vi "Spectrometer Control Panel (No Objects).vi"(8 "error in (no error)":errorcluster) -> (0 "error out":errorcluster)   [LabVIEW 2012]
uses:
  JY-SPEX-TRIAX/controls.llb/Turret Position (TRIAX).ctl
  JY-SPEX-TRIAX/controls.llb/Monochromator System Number.ctl
  JY-SPEX-TRIAX/controls.llb/Mirror Position.ctl
  <vilib>/Utility/error.llb/DialogType.ctl
  JY-SPEX-TRIAX/controls.llb/Slits.ctl
  JY-SPEX-TRIAX/JY-SPEX-TRIAX.lvlib
panel:
  in  "VISA Resource Name":refnum<visa-resource-name>="GPIB0::1::INSTR"
  out "Cluster Out":T4
  in  "Cluster In":T4
  out "?":bool
  out "Title 2":string="Spectrometer Control Program"
  in  "Select Grating":T3
  out "Construct":bool
  out "Init":T5
  out "Status":string
  in  "Shutter":bool
  in  "Set Mirror":bool
  in  "Exit Mirror Pos":bool=TRUE
  in  "Exit":bool
  out "Ready (when flashing)":bool
  out "Slits Open?":bool
  in  "Close Slits":bool
  in  "stepsize":dbl[unit]
  in  "Optimize":bool
  out "groovedensity":dbl[unit] caption="Groove Density"
  out "blazewave":dbl[unit] caption="Blaze Wavelength"
  in  "Set Turret":bool
  out "Title":string="Spectrometer Control Program"
  in  "Reset":bool
  out "Current Wavelength":dbl[unit]
  in  "Target Wavelength":dbl[unit]=4.0000000000000003e-07 min=0.0 max=1.4000000000000001e-06 step=1.0000000000000002e-10
  in  "Jump To Wavelength":bool
  in  "Set Slits":bool
  out "currentlat":dbl[unit] format="%#_6f"
  out "currentaxial":dbl[unit] format="%#_6f"
  in  "gotolat":dbl[unit] min=0.0 max=0.0022 step=1e-05
  in  "gotoaxial":dbl[unit] min=0.0 max=0.0022 step=1e-05 format="%#_6f"
  # "Initialization"
  # "Wavelength Control"
  # "Slit Widths"
  # "Turret and Other Specs"
  # "Target"
  # "Current"
  # "AXIAL/CCD"
  # "LATERAL/PMT"
  # "Axial Entrance"
  # "Lateral Exit"
  # "(will round to nearest step size - 2 µm)"
  # "Grooves/mm       Blaze           Cal Offset\nGrating A           1200           500 nm            -35571\nGrating B           1200           750 nm            -38317\nGrating C             600         1000 nm           -40000 (??)"
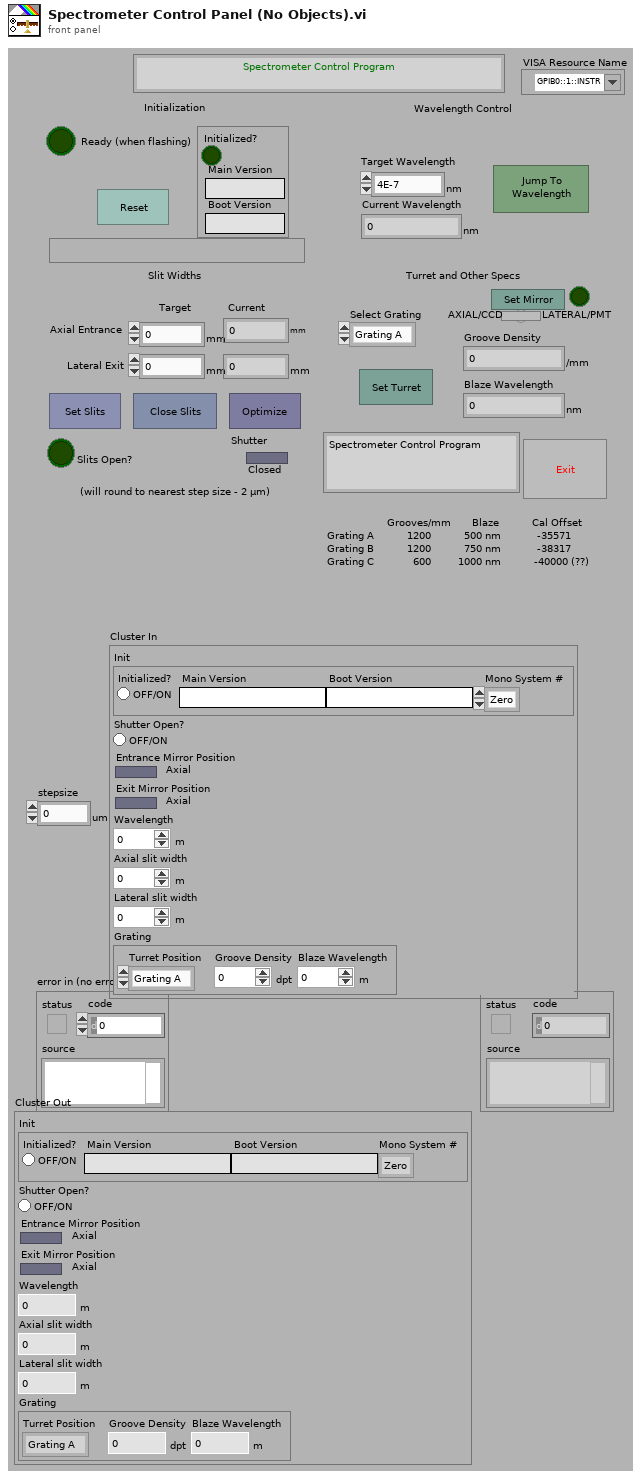
[diagram p1: front panel]
types:
  T1 = typedef "JY-SPEX-TRIAX.lvlib/Monochromator System Number.ctl" = enum16{"Zero", "One"}
  T2 = typedef "JY-SPEX-TRIAX.lvlib/Mirror Position.ctl" = bool
  T3 = typedef "JY-SPEX-TRIAX.lvlib/Turret Position (TRIAX).ctl" = enum16{"Grating A", "Grating B", "Grating C"}
  T4 = cluster{"Init":cluster{"Initialized?":bool, "Main Version":string, "Boot Version":string, "Mono System #":T1}, "Shutter Open?":bool, "Entrance Mirror Position":T2, "Exit Mirror Position":T2, "Wavelength":dbl[unit], "Axial slit width":dbl[unit], "Lateral slit width":dbl[unit], "Grating":cluster{"Turret Position":T3, "Groove Density":dbl[unit], "Blaze Wavelength":dbl[unit]}}
  T5 = cluster{"Initialized?":bool, "Main Version":string, "Boot Version":string, "Spectrometer Number":enum16{"Zero", "One"}}
  T6 = typedef "JY-SPEX-TRIAX.lvlib/Slits.ctl" = enum16{"0 (Front/Axial Entrance)", "1 (Side/Lateral Entrance)", "2 (Front/Axial Exit)", "3 (Side/Lateral Exit)"}
  T7 = typedef "DialogType.ctl" = u16
  T8 = cluster{"Initialized?":bool, "Main Version":string, "Boot Version":string, "Mono System #":T1}
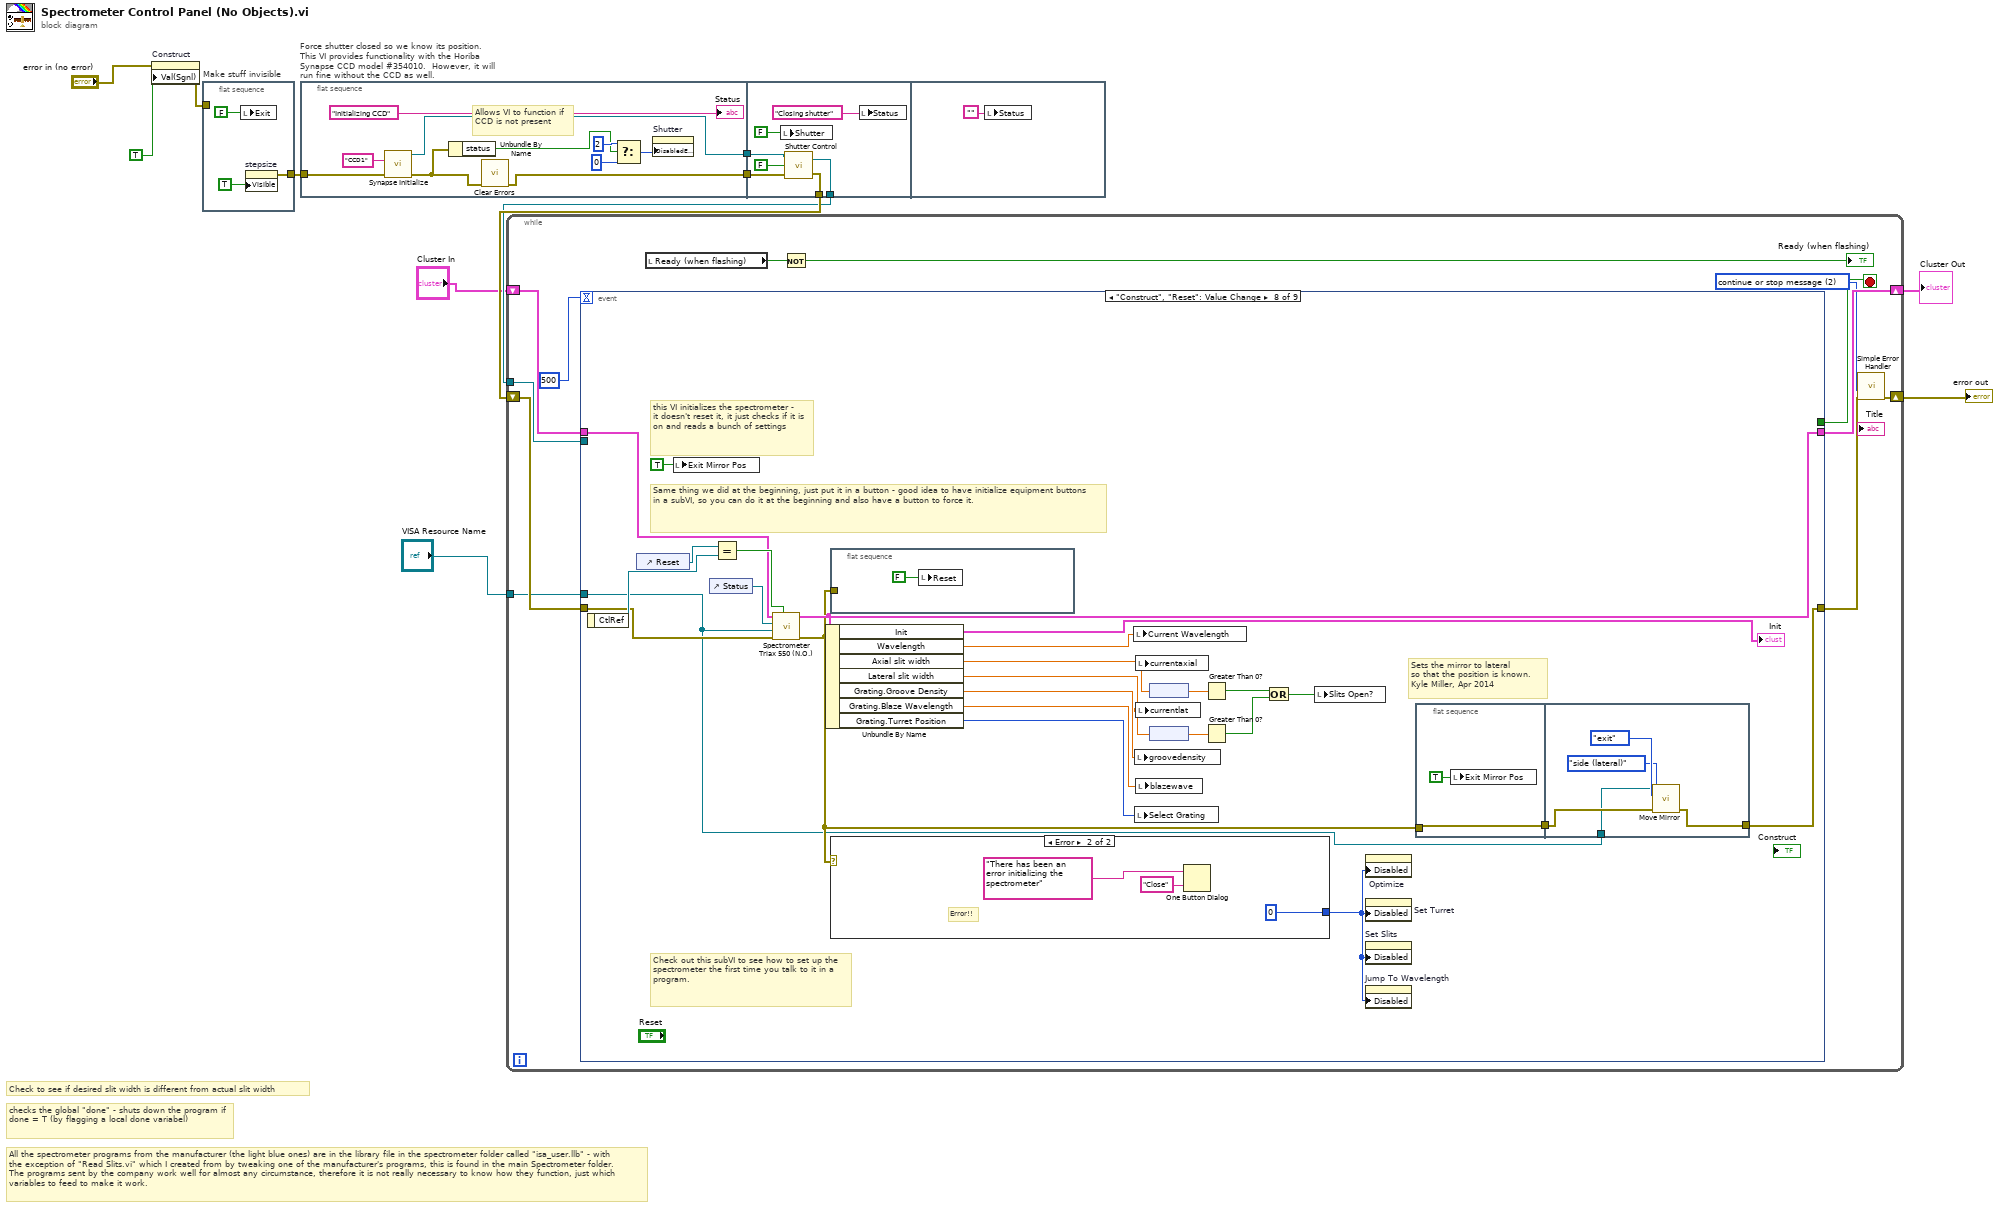
[diagram p0: block diagram]
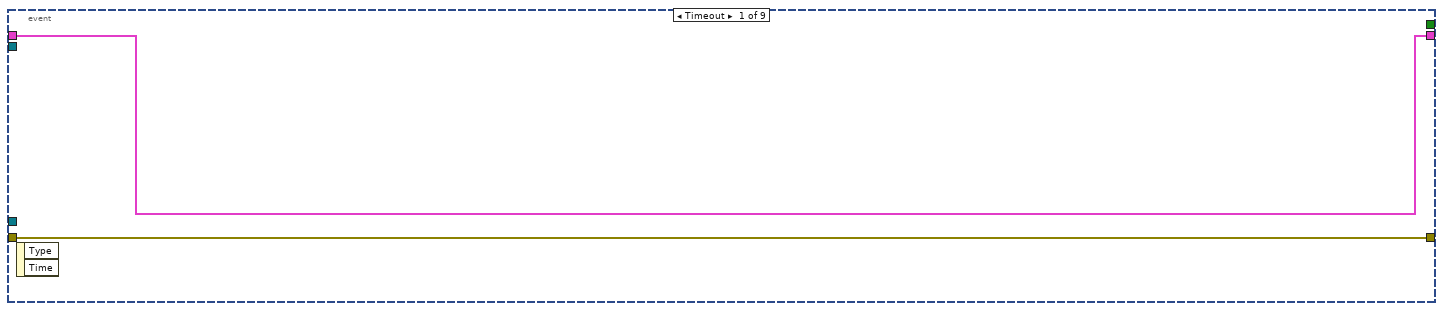
[diagram p2: hidden frame]
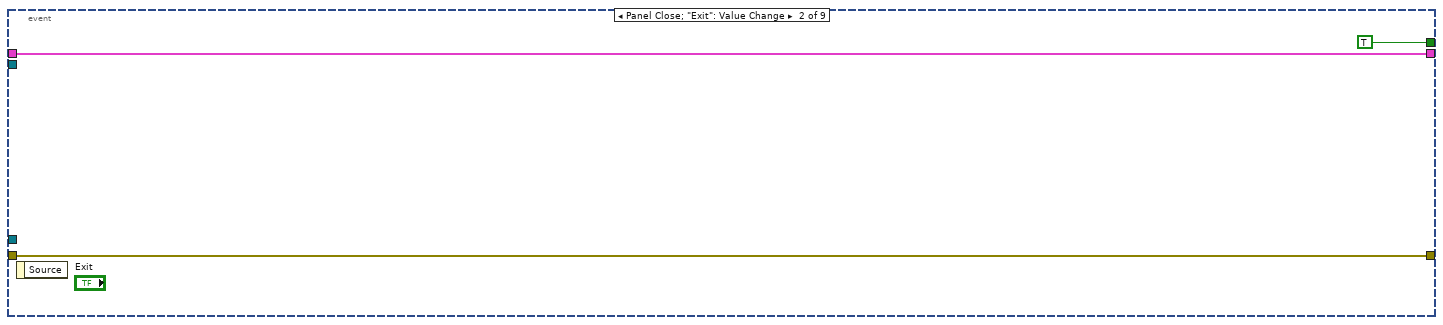
[diagram p3: hidden frame]
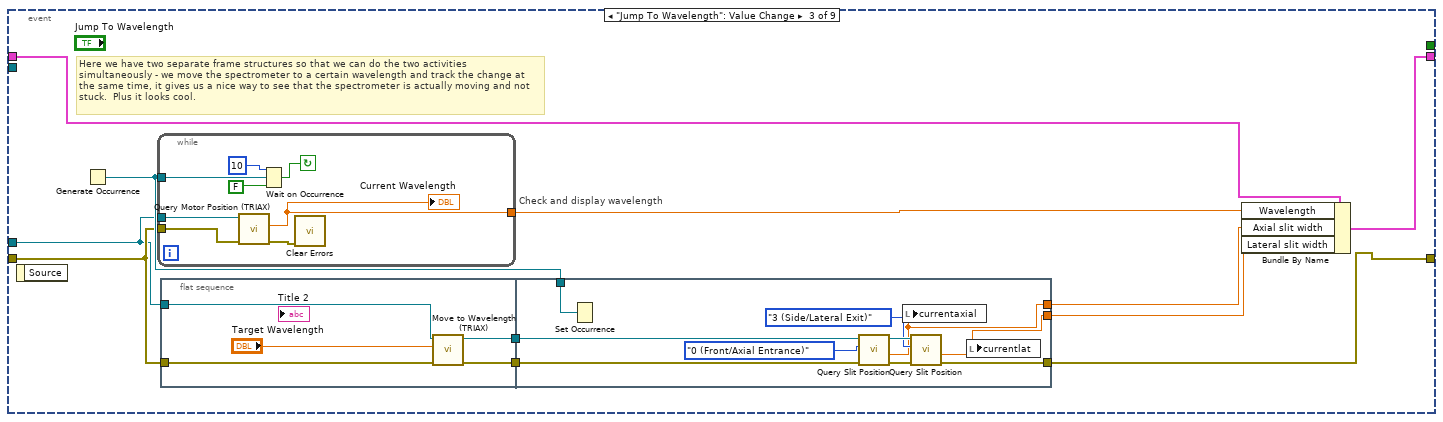
[diagram p4: hidden frame]
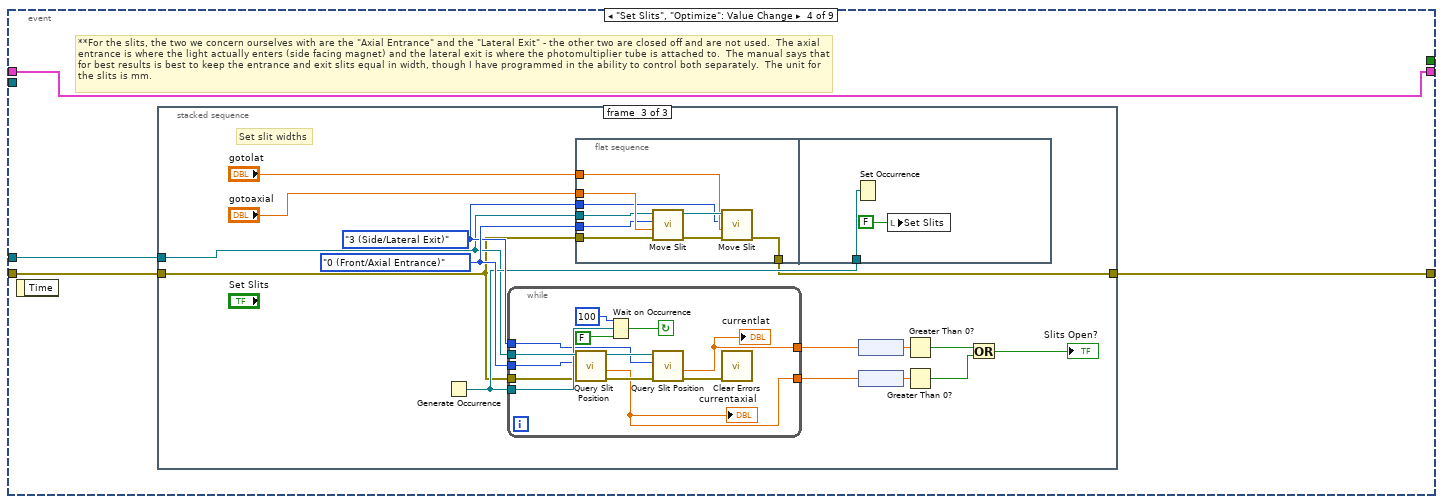
[diagram p5: hidden frame]
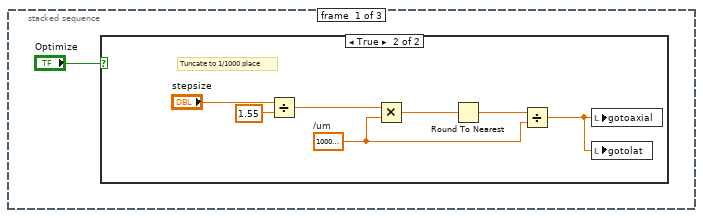
[diagram p6: hidden frame]
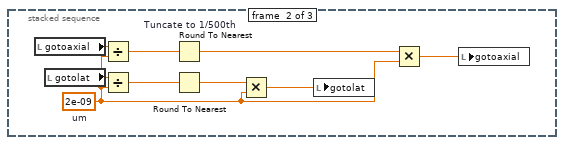
[diagram p8: hidden frame]
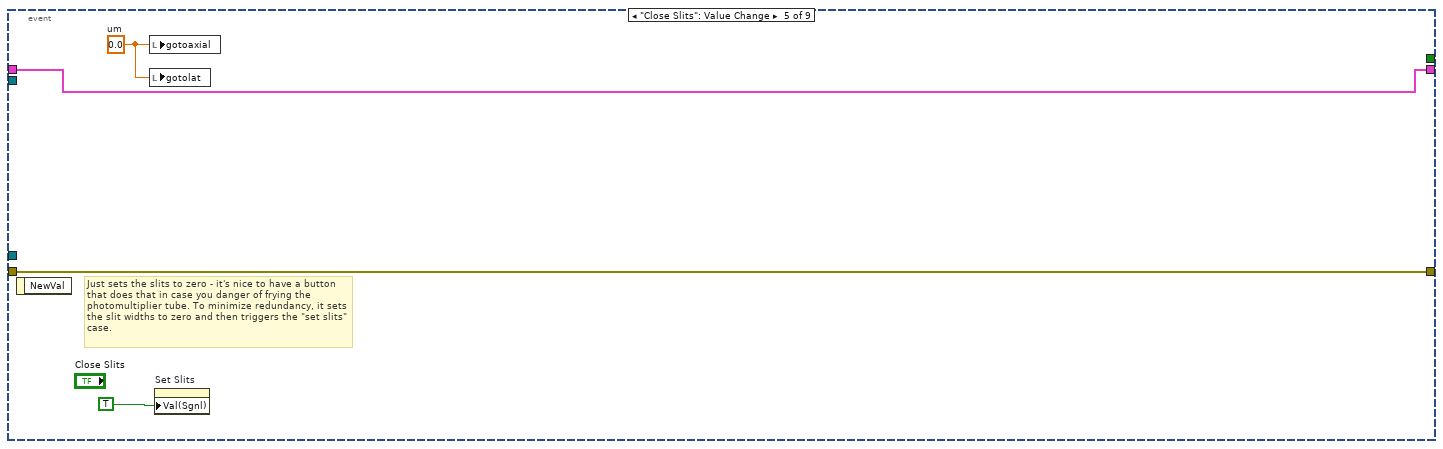
[diagram p9: hidden frame]
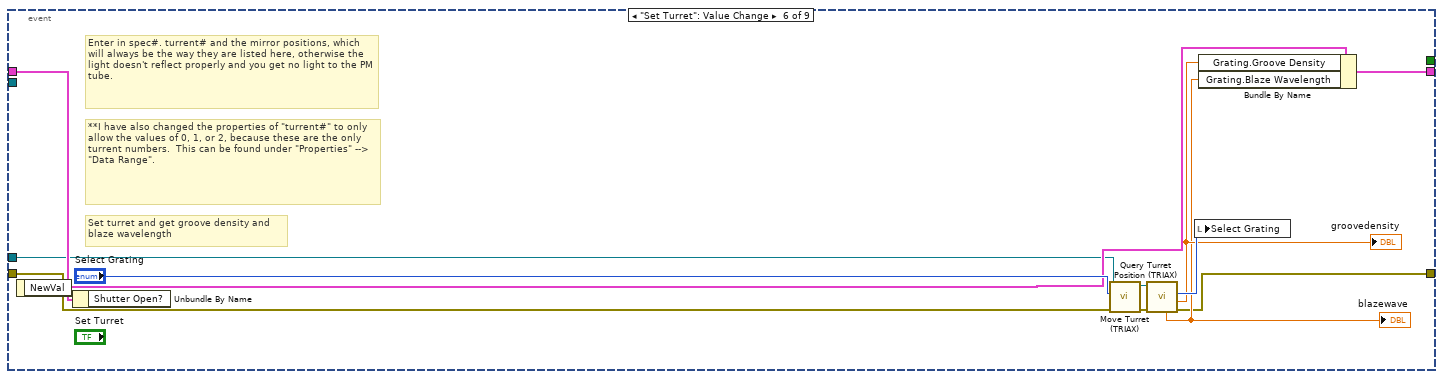
[diagram p10: hidden frame]
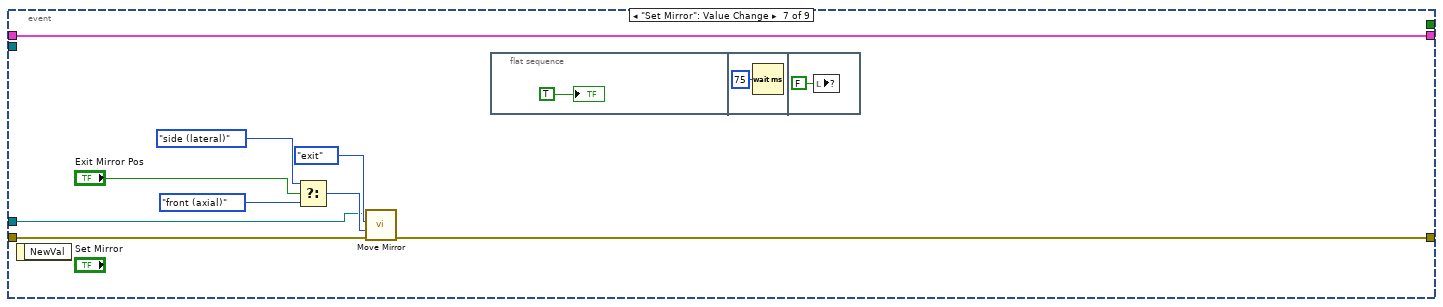
[diagram p11: hidden frame]
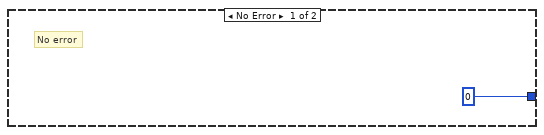
[diagram p12: hidden frame]
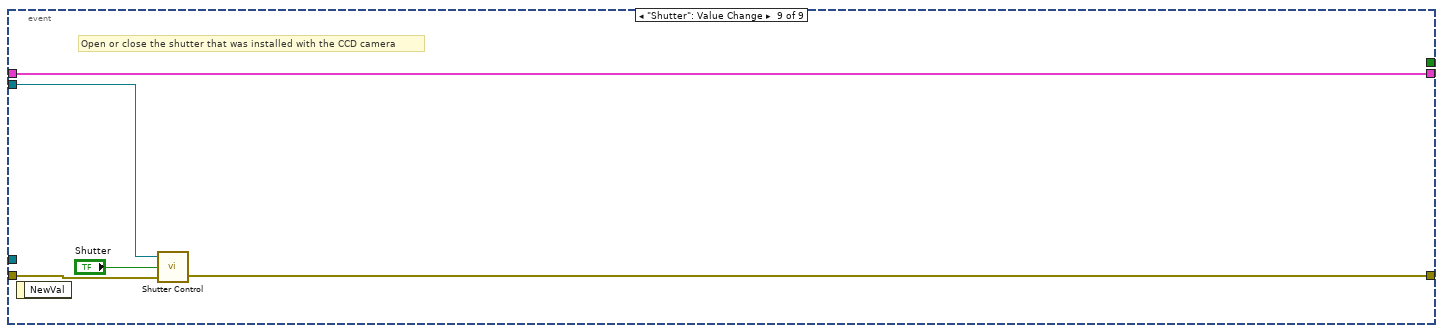
[diagram p13: hidden frame]
diagram:
  # "Check to see if desired slit width is different from actual slit width"
  # "checks the global \"done\" - shuts down the program if done = T (by flagging a local done variabel)"
  # "All the spectrometer programs from the manufacturer (the light blue ones) are in the library file in the spectrometer folder called \"isa_user.llb\" - with the exception of \"Read Slits.vi\" which I created from by tweaking one of the manufacturer's programs, this is found in the main Spectrometer folder.  The programs sent by the company work well for almost any circumstance, therefore it is not really necessary to know how they function, just which variables to feed to make it work."
  n1 = property on="Construct" class="Bool (strict)"(error in="error in (no error)", "Val(Sgnl)"=TRUE ("Value (Signaling)")) -> (error out=w11:errorcluster)  [unwired: 1 in, 1 out]
  n2 = flat-sequence "Make stuff invisible" {
    tunnel: w11 -> [_]
    tunnel: [w14] -> w8
    frame #0 {
      n3 = local write "Exit"(FALSE ("exit")) -> ()
      n4 = property on="stepsize" class="DigNum (strict)"("Visible"=TRUE) -> (error out=w14:errorcluster)  [unwired: 2 in, 1 out]
    }
  }
  n5 = flat-sequence "Force shutter closed so we know its position.  This VI provides functionality with the Horiba Synapse CCD model #354010.  However, it will run fine without the CCD as well." {
    tunnel: w8 -> [w24]
    tunnel: [w18] -> w7
    tunnel: [w22] -> w2
    tunnel: [w30] -> w10
    tunnel: [w29] -> w9
    tunnel: w7 -> [w28]
    tunnel: w2 -> [w27]
    frame #0 {
      # "Allows VI to function if CCD is not present"
      n6 = call "Synapse Initialize.vi"("error in (no error)"=w24, "Unique id"="CCD1") -> ("error out"=w17:errorcluster, "JYCCDLib.IJYCCDReqd"=w22:refnum<k7>)  [unwired: 1 in, 7 out]
      n7 = Unbundle By Name(w17) -> ("status"=w16:bool)
      n8 = call <vilib>:"Clear Errors.vi"("error in (no error)"=w17) -> ("error out"=w18:errorcluster)  [unwired: 6 in]
      n9 = Select(t=2, s=w16, f=0) -> (s? t:f=w19:i32)
      n10 = property on="Shutter" class="Bool (strict)"("DisabledEnum"=w19) -> ()  [unwired: 2 in, 2 out]
      "Status" <- "Initializing CCD" ("initialization progress")
    }
    frame #1 {
      n11 = local write "Shutter"(FALSE ("shutter")) -> ()
      n12 = call "Shutter Control.vi"("input error"=w28, "Shutter"=FALSE, "JYCCDLib.IJYCCDReqd"=w27) -> ("error out"=w30:errorcluster, "JYCCDLib.IJYCCDReqd 2"=w29:refnum<k7>)
      n13 = local write "Status"("Closing shutter" ("initialization progress")) -> ()
    }
    frame #2 {
      n14 = local write "Status"("") -> ()
    }
  }
  n15 = while {
    tunnel: w9 -> [w37]
    shift-right: [w39] -> w3
    shift-left: "Cluster In" -> [w41]
    shift-right: [w36] -> w4
    shift-left: w10 -> [w40]
    tunnel: "VISA Resource Name" -> [w34]
    stop <- w45 stop-if-true
    w35 = T7 2 items=["no dialog", "OK message", "continue or stop message", "OK message + warnings", "continue/stop + warnings"] ("type of dialog (OK msg:1)")
    n16 = event shown="[7] \"Construct\", \"Reset\": Value Change" {
      selector: _ -> [_ _ _ _ _ _ _ _ _]
      dyn-events: _ -> [_ _ _ _ _ _ _ _ _]
      timeout: 500 -> [_ _ _ _ _ _ _ _ _]
      tunnel: [_ TRUE _ _ _ _ _ _ _] -> w45
      tunnel: w37 -> [_ _ _ _ _ _ _ _ w213]
      tunnel: [w46 w49 w51 w86 w147 w159 w160 w184 w211] -> w39
      tunnel: w41 -> [w46 w49 w55 w86 w147 w152 w160 w176 w211]
      tunnel: [w47 w48 w52 w85 w145 w151 w163 w173 w209] -> w38
      tunnel: w40 -> [w47 w48 w54 w87 w145 w150 w162 w177 w210]
      tunnel: w34 -> [_ _ w53 w88 _ w149 w161 w172 _]
      event Timeout {
        n17 = event-data() -> ()  [unwired: 3 out]
      }
      event Panel Close; "Exit": Value Change {
        n18 = event-data() -> ()  [unwired: 2 out]
      }
      event "Jump To Wavelength": Value Change {
        # "Here we have two separate frame structures so that we can do the two activities simultaneously - we move the spectrometer to a certain wavelength and track the change at the same time, it gives us a nice way to see that the spectrometer is actually moving and not stuck.  Plus it looks cool."
        n19 = event-data() -> ()  [unwired: 2 out]
        n20 = Generate Occurrence() -> (w58:refnum<k4>)
        n21 = while "Check and display wavelength" {
          tunnel: [w77] -> w61
          tunnel: w58 -> [w82]
          tunnel: w53 -> [w80]
          tunnel: w54 -> [w78]
          stop <- w84 continue-if-true
          n22 = call "Query Motor Position (TRIAX).vi"("error in (no error)"=w78, "VISA resource name"=w80) -> ("error out"=w79:errorcluster, "wavelength"=w77:dbl[unit])  [unwired: 1 in, 7 out]
          "Current Wavelength" <- w77
          n23 = Wait on Occurrence(1:FALSE ("ignore previous (T)"), 2:w82, 3:10 ("ms timeout (-1)")) -> (0:w84:bool)
          n24 = call <vilib>:"Clear Errors.vi"("error in (no error)"=w79) -> ()  [unwired: 7 out]
        }
        n25 = flat-sequence {
          tunnel: w53 -> [w66]
          tunnel: [w65] -> w57
          tunnel: [w64] -> w56
          tunnel: w54 -> [w63]
          tunnel: [w67] -> w60
          tunnel: [w71] -> w59
          tunnel: w58 -> [w76]
          tunnel: w57 -> [w74]
          tunnel: w56 -> [w73]
          tunnel: [w69] -> w52
          frame #0 {
            n26 = call "Move to Wavelength (TRIAX).vi"("error in (no error)"=w63, "Target wavelength"="Target Wavelength", "VISA resource name"=w66) -> ("error out"=w64:errorcluster, "VISA resource name out"=w65:refnum<visa-resource-name>)  [unwired: 1 in, 6 out]
          }
          frame #1 {
            n27 = Set Occurrence(w76) -> ()
            n28 = call "Query Slit Position.vi"("error in (no error)"=w73, "Slit (Front/Axial Entrance)"=Slits."0 (Front/Axial Entrance)", "VISA resource name"=w74) -> ("error out"=w68:errorcluster, "Slit Position"=w67:dbl[unit], "VISA resource name out"=w75:refnum<visa-resource-name>)  [unwired: 1 in, 5 out]
            n29 = local write "currentaxial"(w67) -> ()
            n30 = call "Query Slit Position.vi"("error in (no error)"=w68, "Slit (Front/Axial Entrance)"=Slits."3 (Side/Lateral Exit)", "VISA resource name"=w75) -> ("error out"=w69:errorcluster, "Slit Position"=w71:dbl[unit])  [unwired: 1 in, 6 out]
            n31 = local write "currentlat"(w71) -> ()
          }
        }
        n32 = Bundle By Name(cluster=w55, "Wavelength"=w61, "Axial slit width"=w60, "Lateral slit width"=w59) -> (w51:T4)
      }
      event "Set Slits", "Optimize": Value Change {
        # "**For the slits, the two we concern ourselves with are the \"Axial Entrance\" and the \"Lateral Exit\" - the other two are closed off and are not used.  The axial entrance is where the light actually enters (side facing magnet) and the lateral exit is where the photomultiplier tube is attached to.  The manual says that for best results is best to keep the entrance and exit slits equal in width, though I have programmed in the ability to control both separately.  The unit for the slits is mm."
        n33 = event-data() -> ()  [unwired: 2 out]
        n34 = stacked-sequence {
          tunnel: [_ _ w108] -> w85
          tunnel: w87 -> [_ _ w106]
          tunnel: w88 -> [_ _ w107]
          frame #0 {
            n35 = case shown="True" "Optimize" {
              frame False {
              }
              frame True {
                w94 = dbl[unit] 1000000000.0  # /um
                # "Tuncate to 1/1000 place"
                n36 = Divide(x="stepsize", y=1.55) -> (x/y=w96:dbl[unit])
                n37 = Multiply(x=w96, y=w94) -> (x*y=w95:dbl)
                n38 = Round To Nearest(number=w95) -> (nearest integer value=w93:dbl)
                n39 = Divide(x=w93, y=w94) -> (x/y=w90:dbl[unit])
                n40 = local write "gotoaxial"(w90) -> ()
                n41 = local write "gotolat"(w90) -> ()
              }
            }
          }
          frame #1 {
            w101 = dbl[unit] 2e-09  # um
            n42 = local read "gotoaxial"() -> (w103:dbl[unit])
            n43 = local read "gotolat"() -> (w102:dbl[unit])
            n44 = Divide(x=w103, y=w101) -> (x/y=w100:dbl)
            n45 = Divide(x=w102, y=w101) -> (x/y=w98:dbl)
            n46 = Round To Nearest "Tuncate to 1/500th"(number=w100) -> (nearest integer value=w99:dbl)
            n47 = Round To Nearest(number=w98) -> (nearest integer value=w97:dbl)
            n48 = Multiply(x=w97, y=w101) -> (x*y=w104:dbl[unit])
            n49 = local write "gotolat"(w104) -> ()
            n50 = Multiply(x=w99, y=w101) -> (x*y=w105:dbl[unit])
            n51 = local write "gotoaxial"(w105) -> ()
          }
          frame #2 {
            w110 = Slits."3 (Side/Lateral Exit)" ("Slit (Front/Axial Entrance)")
            w111 = Slits."0 (Front/Axial Entrance)" ("Slit (Front/Axial Entrance)")
            # "Set slit widths"
            n52 = Generate Occurrence() -> (w109:refnum<k4>)
            n53 = while {
              tunnel: w107 -> [w143]
              tunnel: [w140] -> w113
              tunnel: [w139] -> w112
              tunnel: w109 -> [w138]
              tunnel: w106 -> [w135]
              tunnel: w111 -> [w134]
              tunnel: w110 -> [w133]
              stop <- w136 continue-if-true
              n54 = call "Query Slit Position.vi"("error in (no error)"=w135, "Slit (Front/Axial Entrance)"=w134, "VISA resource name"=w143) -> ("error out"=w142:errorcluster, "Slit Position"=w140:dbl[unit], "VISA resource name out"=w144:refnum<visa-resource-name>)  [unwired: 1 in, 5 out]
              "currentaxial" <- w140
              n55 = Wait on Occurrence(1:FALSE ("ignore previous (T)"), 2:w138, 3:100 ("ms timeout (-1)")) -> (0:w136:bool)
              n56 = call "Query Slit Position.vi"("error in (no error)"=w142, "Slit (Front/Axial Entrance)"=w133, "VISA resource name"=w144) -> ("error out"=w141:errorcluster, "Slit Position"=w139:dbl[unit])  [unwired: 1 in, 6 out]
              "currentlat" <- w139
              n57 = call <vilib>:"Clear Errors.vi"("error in (no error)"=w141) -> ()  [unwired: 7 out]
            }
            n58 = flat-sequence {
              tunnel: "gotoaxial" -> [w128]
              tunnel: "gotolat" -> [w127]
              tunnel: w107 -> [w125]
              tunnel: w106 -> [w124]
              tunnel: w111 -> [w123]
              tunnel: w110 -> [w122]
              tunnel: [w121] -> w108
              tunnel: w109 -> [w131]
              frame #0 {
                n59 = call "Move Slit.vi"("error in (no error)"=w124, "Desired Slit Position"=w128, "Slit (Front/Axial Entrance)"=w123, "VISA resource name"=w125) -> ("error out"=w126:errorcluster, "VISA resource name out"=w129:refnum<visa-resource-name>)  [unwired: 1 in, 5 out]
                n60 = call "Move Slit.vi"("error in (no error)"=w126, "Desired Slit Position"=w127, "Slit (Front/Axial Entrance)"=w122, "VISA resource name"=w129) -> ("error out"=w121:errorcluster)  [unwired: 1 in, 6 out]
              }
              frame #1 {
                n61 = Set Occurrence(w131) -> ()
                n62 = local write "Set Slits"(FALSE ("Move Slits")) -> ()
              }
            }
            n63 = node(w112) -> (w120:dbl)
            n64 = node(w113) -> (w119:dbl)
            n65 = Greater Than 0?(x=w120) -> (x > 0?=w116:bool)
            n66 = Greater Than 0?(x=w119) -> (x > 0?=w117:bool)
            n67 = Or(x=w116, y=w117) -> (x .or. y?=→"Slits Open?":bool)
          }
        }
      }
      event "Close Slits": Value Change {
        w148 = dbl[unit] 0.0  # um
        # "Just sets the slits to zero - it's nice to have a button that does that in case you danger of frying the photomultiplier tube. To minimize redundancy, it sets the slit widths to zero and then triggers the \"set slits\" case."
        n68 = event-data() -> ()  [unwired: 2 out]
        n69 = local write "gotoaxial"(w148) -> ()
        n70 = local write "gotolat"(w148) -> ()
        n71 = property on="Set Slits" class="Bool (strict)"("Val(Sgnl)"=TRUE ("Value (Signaling)")) -> ()  [unwired: 2 in, 2 out]
      }
      event "Set Turret": Value Change {
        # "**I have also changed the properties of \"turrent#\" to only allow the values of 0, 1, or 2, because these are the only turrent numbers.  This can be found under \"Properties\" --> \"Data Range\"."
        # "Enter in spec#. turrent# and the mirror positions, which will always be the way they are listed here, otherwise the light doesn't reflect properly and you get no light to the PM tube."
        # "Set turret and get groove density and \nblaze wavelength"
        n72 = event-data() -> ()  [unwired: 2 out]
        n73 = Unbundle By Name(w152) -> ()  [unwired: 1 out]
        n74 = call "Move Turret (TRIAX).vi"("error in (no error)"=w150, "turret position (0)"="Select Grating", "VISA resource name"=w149) -> ("error out"=w156:errorcluster, "VISA resource name out"=w157:refnum<visa-resource-name>)  [unwired: 1 in, 6 out]
        n75 = call "Query Turret Position (TRIAX).vi"("error in (no error)"=w156, "VISA resource name"=w157) -> ("error out"=w151:errorcluster, "Groove Density"=w154:dbl[unit], "Turret Position"=w155:T3, "Blaze Wavelength"=w153:dbl[unit])  [unwired: 1 in, 5 out]
        "blazewave" <- w153
        "groovedensity" <- w154
        n76 = local write "Select Grating"(w155) -> ()
        n77 = Bundle By Name(cluster=w152, "Grating.Groove Density"=w154, "Grating.Blaze Wavelength"=w153) -> (w159:T4)
      }
      event "Set Mirror": Value Change {
        n78 = event-data() -> ()  [unwired: 2 out]
        n79 = Select(t=enum16{"side (lateral)", "front (axial)"}."side (lateral)" ("position (side/lateral)"), s="Exit Mirror Pos", f=enum16{"side (lateral)", "front (axial)"}."front (axial)" ("position (side/lateral)")) -> (s? t:f=w164:enum16{"side (lateral)", "front (axial)"})
        n80 = call "Move Mirror.vi"("error in (no error)"=w162, "position (side/lateral)"=w164, "mirror (exit)"=enum16{"entrance", "exit"}."exit", "VISA resource name"=w161) -> ("error out"=w163:errorcluster)  [unwired: 1 in, 6 out]
        n81 = flat-sequence {
          frame #0 {
            "?" <- TRUE ("Mirror set")
          }
          frame #1 {
            n82 = Wait (ms)(milliseconds to wait=u32 75) -> ()  [unwired: 1 out]
          }
          frame #2 {
            n83 = local write item#29(FALSE ("Mirror set")) -> ()
          }
        }
      }
      event "Construct", "Reset": Value Change {
        # "Sets the mirror to lateral\nso that the position is known.\nKyle Miller, Apr 2014"
        # "Check out this subVI to see how to set up the spectrometer the first time you talk to it in a program."
        # "this VI initializes the spectrometer - it doesn't reset it, it just checks if it is on and reads a bunch of settings"
        # "Same thing we did at the beginning, just put it in a button - good idea to have initialize equipment buttons in a subVI, so you can do it at the beginning and also have a button to force it."
        n84 = event-data() -> ("CtlRef"=w180:refnum<vi>)  [unwired: 1 out]
        n85 = control-ref of="Reset"() -> (w179:refnum<vi>)
        n86 = local write "Exit Mirror Pos"(TRUE ("Exit Mirror Pos")) -> ()
        n87 = control-ref of="Status"() -> (w182:refnum<vi>)
        n88 = Equal?(x=w179, y=w180) -> (x = y?=w178:bool)
        n89 = call "Spectrometer Triax 550 (N.O.).vi"("Force Reset? (F)"=w178, "error in (no error)"=w177, "VISA Resource Name"=w172, "Ref to a Status Box"=w182, "Cluster In"=w176) -> ("error out"=w174:errorcluster, "Cluster Out"=w184:T4)  [unwired: 5 in]
        n90 = Unbundle By Name(w184) -> ("Init"=→"Init":T8, "Wavelength"=w192:dbl[unit], "Axial slit width"=w185:dbl[unit], "Lateral slit width"=w189:dbl[unit], "Grating.Groove Density"=w191:dbl[unit], "Grating.Blaze Wavelength"=w190:dbl[unit], "Grating.Turret Position"=w183:T3)
        n91 = flat-sequence {
          tunnel: w174 -> [_]
          frame #0 {
            n92 = local write "Reset"(FALSE ("initialize")) -> ()
          }
        }
        n93 = case shown="Error" w174 {
          tunnel: [0 0] -> w196
          frame No Error {
            # "No error"
          }
          frame Error {
            # "Error!!"
            n94 = One Button Dialog(message="There has been an error initializing the spectrometer", button name ("OK")="Close") -> ()  [unwired: 1 out]
          }
        }
        n95 = local write "Current Wavelength"(w192) -> ()
        n96 = local write "groovedensity"(w191) -> ()
        n97 = local write "Select Grating"(w183) -> ()
        n98 = local write "currentaxial"(w185) -> ()
        n99 = local write "currentlat"(w189) -> ()
        n100 = local write "blazewave"(w190) -> ()
        n101 = node(w185) -> (w187:dbl)
        n102 = node(w189) -> (w186:dbl)
        n103 = Greater Than 0?(x=w187) -> (x > 0?=w195:bool)
        n104 = Greater Than 0?(x=w186) -> (x > 0?=w194:bool)
        n105 = Or(x=w195, y=w194) -> (x .or. y?=w193:bool)
        n106 = local write "Slits Open?"(w193) -> ()
        n107 = property on="Optimize" class="Bool"("Disabled"=w196) -> ()  [unwired: 2 in, 2 out]
        n108 = property on="Set Turret" class="Bool"("Disabled"=w196) -> ()  [unwired: 2 in, 2 out]
        n109 = property on="Set Slits" class="Bool (strict)"("Disabled"=w196) -> ()  [unwired: 2 in, 2 out]
        n110 = property on="Jump To Wavelength" class="Bool"("Disabled"=w196) -> ()  [unwired: 2 in, 2 out]
        n111 = flat-sequence {
          tunnel: w174 -> [w197]
          tunnel: [w197] -> w175
          tunnel: w175 -> [w201]
          tunnel: [w200] -> w173
          tunnel: w172 -> [w199]
          frame #0 {
            n112 = local write "Exit Mirror Pos"(TRUE ("Exit Mirror Pos")) -> ()
          }
          frame #1 {
            n113 = call "Move Mirror.vi"("error in (no error)"=w201, "position (side/lateral)"=enum16{"side (lateral)", "front (axial)"}."side (lateral)", "mirror (exit)"=enum16{"entrance", "exit"}."exit", "VISA resource name"=w199) -> ("error out"=w200:errorcluster)  [unwired: 1 in, 6 out]
          }
        }
      }
      event "Shutter": Value Change {
        # "Open or close the shutter that was installed with the CCD camera"
        n114 = event-data() -> ()  [unwired: 2 out]
        n115 = call "Shutter Control.vi"("input error"=w210, "Shutter"="Shutter", "JYCCDLib.IJYCCDReqd"=w213) -> ("error out"=w209:errorcluster)  [unwired: 1 out]
      }
    }
    n116 = local read "Ready (when flashing)"() -> (w43:bool)
    n117 = Not(x=w43) -> (.not. x?=→"Ready (when flashing)":bool)
    n118 = call <vilib>:"Simple Error Handler.vi"("type of dialog (OK msg:1)"=w35, "error in (no error)"=w38) -> ("error out"=w36:errorcluster)  [unwired: 7 out]
  }
  "error out" <- w4
  "Cluster Out" <- w3
